vi "FdxCmdTxUDPWriteCvi.vi"(6 "ByteCount":i32=-1, 8 "error in":errorcluster, 9 "Data":u8[](array[numeric]), 10 "UdpHandle":u32, 11 "InstrumentHandle":u32) -> (0 "error out":errorcluster, 1 "BytesWritten":u32, 2 "UdpHandleOut":u32, 3 "InstrumentHandle":u32)   [LabVIEW 2020, in "AIM664LV.lvlib"]
doc: "This function is used to write a pure message to a UDP port. This port can be a sampling or a queuing port. If the data size is not applicable for the data size associated to this port, this function will return an error.\nFor sampling ports this function initializes / modifies data contents.\nFor queuing ports a transmission is initiated when data is written to a UDP port.\nThis function can be used if the transmitter is running or not running.\nFor sampling ports this function should be called before the port is started to initialize the data contents of the sampling port."
uses:
  AIM664LV.lvlib
  AFDX_LibraryAdmin/FdxGlobalDllPath.vi
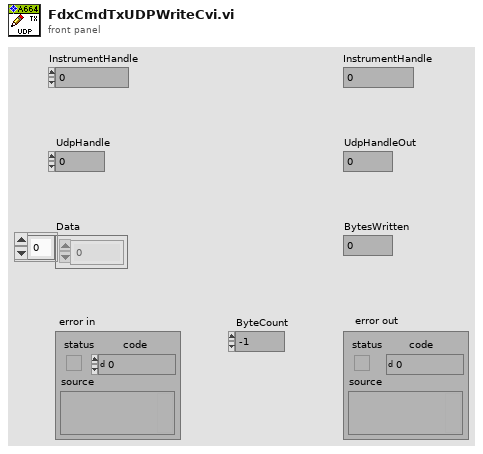
[diagram p1: front panel]
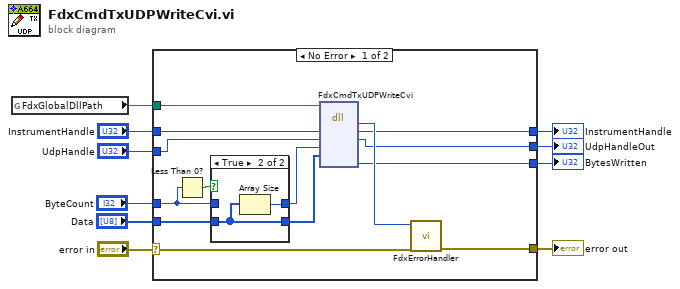
[diagram p0: block diagram]
diagram:
  n1 = global read "FdxGlobalDllPath.vi" "FdxGlobalDllPath"() -> (w8:path)
  n2 = case shown="No Error" "error in" {
    selector: "error in" -> [w23 w31]
    tunnel: [w24 w31] -> w10
    tunnel: w8 -> [w21 _]
    tunnel: "InstrumentHandle" -> [w20 w30]
    tunnel: [w19 w30] -> w6
    tunnel: [w18 _] -> w5
    tunnel: "UdpHandle" -> [w11 w29]
    tunnel: [w17 w29] -> w3
    tunnel: "Data" -> [w15 _]
    tunnel: "ByteCount" -> [w13 _]
    frame No Error {
      n3 = Less Than 0?(x=w13) -> (x < 0?=w16:bool)
      n4 = case shown="True" w16 {
        tunnel: w15 -> [w25 w27]
        tunnel: w13 -> [w26 _]
        tunnel: [w26 w28] -> w12
        tunnel: [w25 w27] -> w14
        frame False {
        }
        frame True {
          n5 = Array Size(array=w27) -> (size(s)=w28:i32)
        }
      }
      n6 = dll-call lib="aim_fdx.19.dll" fn="FdxCmdTxUDPWriteCvi"(path in=w21, "InstrumentHandle"=w20, "UdpHandle"=w11, "ByteCount"=w12, "Data"=w14) -> ("status"=w22:i32, "InstrumentHandle"=w19:u32, "UdpHandle"=w17:u32, "BytesWritten"=w18:u32)  [unwired: 4 in, 3 out]
      n7 = call "FdxErrorHandler.vi"("error in"=w23, "AIM Error"=w22) -> ("error out"=w24:errorcluster)  [unwired: 9 in]
    }
    frame Error {
    }
  }
  "error out" <- w10
  "InstrumentHandle" <- w6
  "BytesWritten" <- w5
  "UdpHandleOut" <- w3
